vi "PH_SHS_Analysis_Calibrator.constructor.vi"(0 "name":string, 2 "data in":string, 5 "error in":errorcluster) -> (14 "i ref out":refnum<vi>, 16 "data out":string, 19 "error out":errorcluster)   [LabVIEW 2014, in "PH_SHS_Analysis_Calibrator.lvlib"]
doc: "This class takes and stores several beam profile settings. This is relevant for the class PH_ImageOperator.\n\nThis class is part of the PHELIX user layer.\n\nauthor: Stefan Götte, GSI\n\nLicense Agreement for this software:\n\nCopyright (C)\nGesellschaft für Schwerionenforschung, GSI\nPlanckstr. 1\n64291 Darmstadt\nGermany\n\nContact: D.Beck@gsi.de \n\nThis program is free software; you can redistribute it and/or modify it under the terms of the \nGNU General Public License as published by the Free Software Foundation; either version 2 of \nthe license, or (at your option) any later version.\n\nThis program is distributed in the hope that it will be useful, but WITHOUT ANY WARRANTY; \nwithout even the implied warranty of MERCHANTABILITY or FITNESS FOR A PARTICULAR PURPOSE. See the GNU General License for more details (http://www.gnu.org).\n\nGesellschaft für Schwerionenforschung, GSI\nPlanckstr. 1, 64291 Darmstadt, Germany\nFor all questions and ideas contact: M.Richter@gsi.de, H.Brand@gsi.de or D.Beck@gsi.de.\nLast update: 16-JUN-2004"
uses:
  PH_SHS_Analysis_Calibrator.lvlib
  PH_Img_BaseClass/PH_Img_BaseClass.Palette.ctl
  CSCore/CSObj/CSObj.lvlib
  PH_Img_BaseClass/PH_Img_BaseClass.lvlib
  PH_Common/PH_Common.lvlib
  PH_Class/PH_Class.lvlib
  PH_SM_Class/PH_SM_Class.lvlib
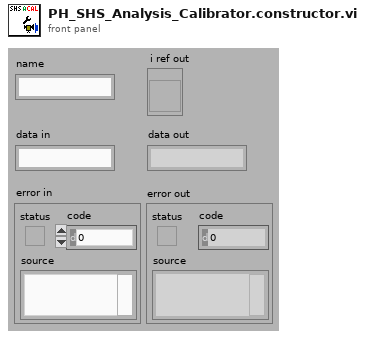
[diagram p1: front panel]
types:
  T1 = enum16{"SetAttribute", "GetAttribute", "CreateAttribute", "DestroyAttribute", "DestroyAllAtributes"}
  T2 = typedef "PH_Img_BaseClass.lvlib/PH_Img_BaseClass.Palette.ctl" = i32
  T3 = typedef "PH_SHS_Analysis_Calibrator.lvlib/PH_SHS_Analysis_Calibrator.i attribute.ctl" = cluster{"GUI Refs":cluster{"Available Cams":refnum<vi>, "OK":refnum<vi>, "Skip":refnum<vi>, "Repeat":refnum<vi>, "Cancel":refnum<vi>, "Dialog":refnum<vi>, "Enough Images?":refnum<vi>}, "Cam instances":string[], "Status":cluster{"#":i32, "Data calculated":bool, "Wanted #":i32}, "IMAQ Image Array":T4[], "Pixel Size [µm]":dbl, "MLA Pitch [µm]":dbl, "Method":enum16{"automatic", "manual"}, "Enough Images?":bool, "SHS Reference Result":T5, "Calculation Error":errorcluster}
  T4 = typedef "IMAQ Image.ctl" = refnum<image>
  T5 = typedef "SHS_Common.lvlib/SHSReference.ctl" = cluster{"Reference":T6[][], "Lens Array Pitch [px]":dbl}
  T6 = typedef "SHS_Common.lvlib/ReferencePoint.ctl" = cluster{"Rect":T7, "Point":T8}
  T7 = typedef "SHS_Common.lvlib/Rectangle.ctl" = cluster{"Left":i32, "Top":i32, "Right":i32, "Bottom":i32}
  T8 = typedef "SHS_Common.lvlib/Point.ctl" = cluster{"x":dbl, "y":dbl, "valid?":bool, "weight":dbl}
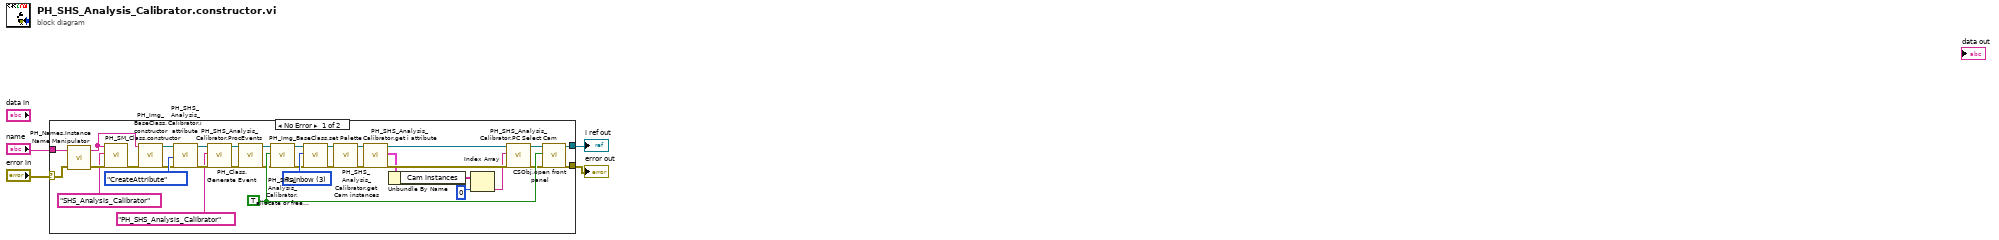
[diagram p0: block diagram]
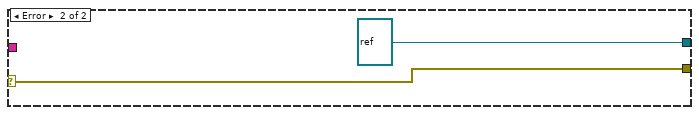
[diagram p2: hidden frame]
diagram:
  n1 = case shown="No Error" "error in" {
    selector: "error in" -> [w32 w39]
    tunnel: "name" -> [w33 _]
    tunnel: [w36 refnum<vi> refnum ("i ref out")] -> w3
    tunnel: [w35 w39] -> w2
    frame No Error {
      w34 = T2 3 items=["Grey", "Binary", "Gradient", "Rainbow", "Temperature"] ("Palette")
      w37 = TRUE ("front panel open")
      n2 = call "PH_Names.Instance Name Manipulator.vi"("error in (no error)"=w32, "name in"=w33) -> ("error out"=w24:errorcluster, "name out"=w22:string)  [unwired: 1 in, 1 out]
      n3 = call "PH_SM_Class.constructor.vi"("name"=w22, "data in"="SHS_Analysis_Calibrator" ("object"), "error in"=w24) -> ("error out"=w23:errorcluster)  [unwired: 14 in, 2 out]
      n4 = call "PH_Img_BaseClass.constructor.vi"("name"=w22, "error in(no error)"=w23) -> ("i ref out"=w31:refnum<vi>, "error out"=w30:errorcluster)  [unwired: 15 in, 1 out]
      n5 = call "PH_SHS_Analysis_Calibrator.i attribute.vi"("VI Refnum"=w31, "Action"=T1."CreateAttribute", "error in (no error)"=w30) -> ("VI Refnum out"=w29:refnum<vi>, "error out"=w28:errorcluster)  [unwired: 14 in, 1 out]
      n6 = call "PH_Class.Generate Event.vi"("i ref in"=w29, "Class"="PH_SHS_Analysis_Calibrator", "error in (no error)"=w28) -> ("i ref out"=w19:refnum<vi>, "error out"=w20:errorcluster)  [unwired: 15 in]
      n7 = call "PH_SHS_Analysis_Calibrator.ProcEvents.vi"("i ref in"=w19, "error in"=w20) -> ("i ref out"=w26:refnum<vi>, "error out"=w25:errorcluster)  [unwired: 16 in]
      n8 = call "PH_SHS_Analysis_Calibrator.allocate or free img space.vi"("i ref in"=w26, "Allocate?"=w37, "error in (no error)"=w25) -> ("i ref out"=w18:refnum<vi>, "error out"=w17:errorcluster)  [unwired: 15 in]
      n9 = call "PH_Img_BaseClass.set Palette.vi"("i ref in"=w18, "Palette"=w34, "error in (no error)"=w17) -> ("i ref out"=w6:refnum<vi>, "error out"=w5:errorcluster)  [unwired: 15 in]
      n10 = call "PH_SHS_Analysis_Calibrator.get Cam instances.vi"("i ref in"=w6, "error in"=w5) -> ("i ref out"=w9:refnum<vi>, "error out"=w10:errorcluster)  [unwired: 16 in]
      n11 = call "PH_SHS_Analysis_Calibrator.get i attribute.vi"("i ref in"=w9, "error in (no error)"=w10) -> ("i ref out"=w15:refnum<vi>, "i attribute"=w11:T3, "error out"=w16:errorcluster)  [unwired: 15 in]
      n12 = Unbundle By Name(w11) -> ("Cam instances"=w12:string[])
      n13 = Index Array(array=w12, index=0) -> (element=w14:string)
      n14 = call "PH_SHS_Analysis_Calibrator.PC Select Cam.vi"("VI in"=w15, "Source"=w14, "error in (no error)"=w16) -> ("VI out"=w8:refnum<vi>, "error out"=w7:errorcluster)  [unwired: 15 in]
      n15 = call "CSObj.open front panel.vi"("i ref in"=w8, "frontPanelOpen"=w37, "error in (no error)"=w7) -> ("i ref out"=w36:refnum<vi>, "error out"=w35:errorcluster)  [unwired: 15 in]
    }
    frame Error {
    }
  }
  "i ref out" <- w3
  "error out" <- w2
